vi "aft_check_real_waveform_fs_consistency_sub.vi"(7 "init":bool, 8 "error in (no error)":errorcluster, 9 "dt in":dbl, 10 "signal in 2":waveform(dbl), 11 "signal in 1":waveform(dbl)) -> (0 "error out":errorcluster, 1 "dt out":dbl)   [LabVIEW 2017, in "NI_AdaptiveFilter.lvlib"]
doc: "To check waveform sampling interval consistency."
uses:
  <vilib>/addons/Adaptive Filters/NI_AdaptiveFilter.lvlib
  <vilib>/addons/Adaptive Filters/Utilities/AFT Errors.ctl
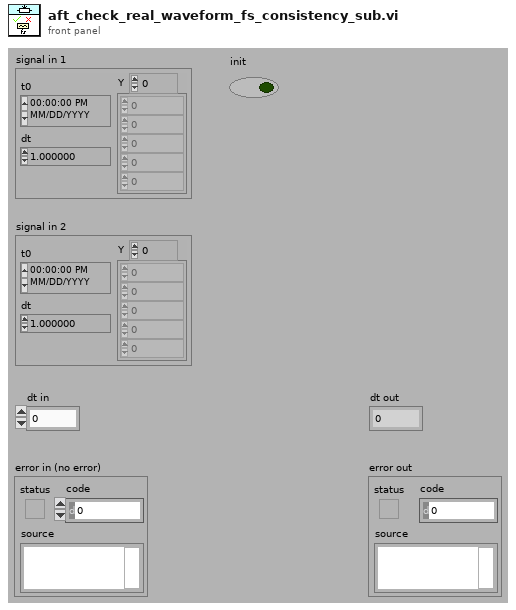
[diagram p1: front panel]
types:
  T1 = typedef "NI_AdaptiveFilter.lvlib/AFT Errors.ctl" = i32
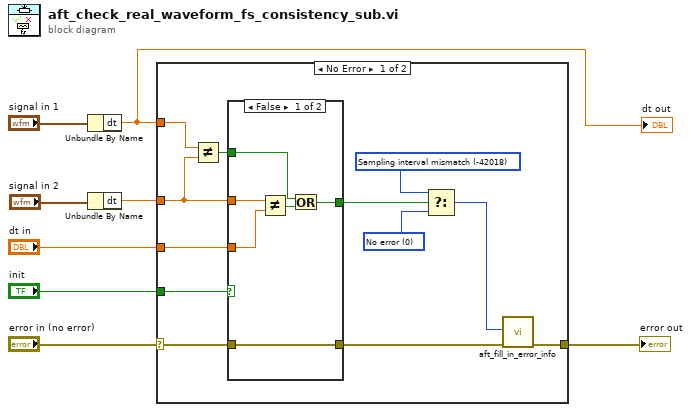
[diagram p0: block diagram]
diagram:
  n1 = Unbundle By Name("signal in 1") -> ("dt"=w2:dbl)
  "dt out" <- w2
  n2 = Unbundle By Name("signal in 2") -> ("dt"=w3:dbl)
  n3 = case shown="No Error" "error in (no error)" {
    selector: "error in (no error)" -> [w9 w29]
    tunnel: "init" -> [w19 _]
    tunnel: [w12 w29] -> w7
    tunnel: "dt in" -> [w20 _]
    tunnel: w2 -> [w17 _]
    tunnel: w3 -> [w16 _]
    frame No Error {
      w11 = T1 -42018 items=["No error"=0, "Sampling interval mismatch"=-42018, "Invalid FPGA target"=-42150, "Invalid filter configurations"=-42151, "LabVIEW FPGA or NI-RIO not installed"=-42152, "Fail to overwrite"=-42153, "File exists in memory"=-42154] ("AFT errors")
      w10 = T1 0 items=["No error"=0, "Sampling interval mismatch"=-42018, "Invalid FPGA target"=-42150, "Invalid filter configurations"=-42151, "LabVIEW FPGA or NI-RIO not installed"=-42152, "Fail to overwrite"=-42153, "File exists in memory"=-42154] ("AFT errors")
      n4 = Not Equal?(x=w17, y=w16) -> (x != y?=w18:bool)
      n5 = case shown="False" w19 {
        tunnel: w20 -> [w21 _]
        tunnel: w9 -> [w22 w27]
        tunnel: w18 -> [w25 w28]
        tunnel: w16 -> [w26 _]
        tunnel: [w23 w28] -> w14
        tunnel: [w22 w27] -> w13
        frame False {
          n6 = Not Equal?(x=w26, y=w21) -> (x != y?=w24:bool)
          n7 = Or(x=w25, y=w24) -> (x .or. y?=w23:bool)
        }
        frame True {
        }
      }
      n8 = Select(t=w11, s=w14, f=w10) -> (s? t:f=w15:T1)
      n9 = call <vilib>:"aft_fill_in_error_info.vi"("error in"=w13, "status code"=w15) -> ("error out"=w12:errorcluster)  [unwired: 2 in, 7 out]
    }
    frame Error {
    }
  }
  "error out" <- w7
